vi "读取data.vi"(8 "error in (no error)":errorcluster caption="错误输入（无错误）", 11 "LS-H600-TCP Client输入":refnum<class "LS-H600-TCP Client.lvclass">) -> (0 "error out":errorcluster caption="错误输出", 2 "data":T1, 3 "LS-H600-TCP Client输出":refnum<class "LS-H600-TCP Client.lvclass">)   [LabVIEW 2022 SP3, in "LS-H600-TCP Client.lvlib" / "LS-H600-TCP Client.lvclass"]
uses:
  LS-H600-TCP Client.lvclass
  LS-H600-TCP Client.lvclass/LS-H600-TCP Client.ctl
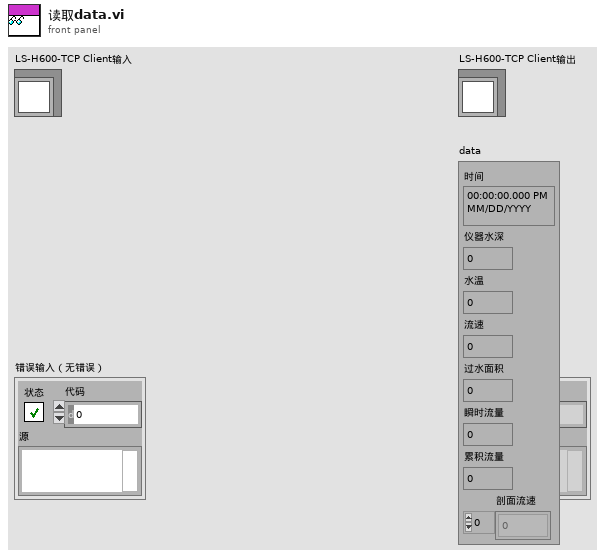
[diagram p1: front panel]
types:
  T1 = cluster{"时间":timestamp, "仪器水深":dbl, "水温":dbl, "流速":dbl, "过水面积":dbl, "瞬时流量":dbl, "累积流量":dbl, "剖面流速":dbl[]}
  T2 = cluster{"数据输出":string, "data":cluster{"时间":timestamp, "仪器水深":dbl, "水温":dbl, "流速":dbl, "过水面积":dbl, "瞬时流量":dbl, "累积流量":dbl, "剖面流速":dbl[]}, "连接错误":errorcluster}
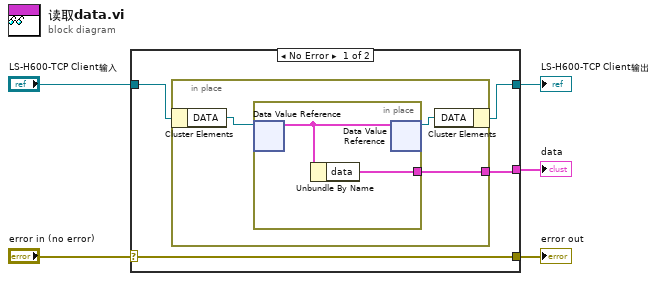
[diagram p0: block diagram]
diagram:
  n1 = case shown="No Error" "error in (no error)" {
    selector: "error in (no error)" -> [w9 w15]
    tunnel: [w9 w15] -> w4
    tunnel: [w7 w16] -> w2
    tunnel: "LS-H600-TCP Client输入" -> [w8 w16]
    tunnel: [w6 _] -> w1
    frame No Error {
      n2 = in-place {
        in-place-border: [w10] -> w6
        n3 = in-place-cluster #1(w8) -> ("DATA"=w12:refnum<data-value>)
        n4 = in-place {
          in-place-border: [w13] -> w10
          n5 = in-place-dvr #2(w12) -> (w14:T2)  [unwired: 1 out]
          n6 = Unbundle By Name(w14) -> ("data"=w13:T1)
          n7 = in-place-dvr #2(w14) -> (w11:refnum<data-value>)  [unwired: 1 out]
        }
        n8 = in-place-cluster #1("DATA"=w11) -> (w7:refnum<class "LS-H600-TCP Client.lvclass">)
      }
    }
    frame Error {
    }
  }
  "error out" <- w4
  "LS-H600-TCP Client输出" <- w2
  "data" <- w1
